vi "Autoshift.vi"() -> ()   [LabVIEW 2017]
uses:
  <vilib>/Rock Robotics/WPI/Solenoid/WPI_SolenoidDevRef.ctl
  <vilib>/Rock Robotics/WPI/Solenoid/WPI_SolenoidChannel.ctl
  <vilib>/Rock Robotics/WPI/Solenoid/WPI_SolenoidValue.ctl
  <vilib>/Rock Robotics/WPI/ThirdParty/Sensors/navX/_TypeDefs/FRIC_navX_DeviceNumbersTypeDef.ctl
  <vilib>/Rock Robotics/WPI/Utilities/WPI_GetSetVariantRefNum.vi
  <vilib>/Rock Robotics/WPI/ThirdParty/Phoenix-LabVIEW/Motor Controller/Get/CTRE_Phoenix_MotorController_GetSelectedSensorData.vi
panel:
  in  "refnum name 3":string="My Motor RefNum"
  in  "refnum name 2":string="My Motor RefNum"
  in  "refnum name":string="My Joystick RefNum"
  in  "ShifterRef":T1={"DevStatus"={"status"=FALSE, "code"=0, "source"=""}, "Pneumatics Control Module"=0, "Forward Solenoid Channel"=enum."Invalid", "Reverse Solenoid Channel"=enum."Invalid"}
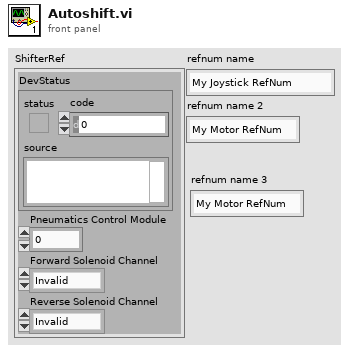
[diagram p1: front panel]
types:
  T1 = typedef "WPI_SolenoidDevRef.ctl" = cluster{"DevStatus":errorcluster, "Pneumatics Control Module":u8, "Forward Solenoid Channel":T2, "Reverse Solenoid Channel":T2}
  T2 = typedef "WPI_SolenoidChannel.ctl" = enum8{"Solenoid 0", "Solenoid 1", "Solenoid 2", "Solenoid 3", "Solenoid 4", "Solenoid 5", "Solenoid 6", "Solenoid 7", "Invalid"}
  T3 = typedef "FRIC_navX_DeviceNumbersTypeDef.ctl" = enum16{"Dev0", "Dev1", "Dev2", "Dev3"}
  T4 = typedef "WPI_SolenoidValue.ctl" = enum16{"Off", "On", "Forward", "Reverse"}
  T5 = typedef "WPI_MotorControlDeviceRef.ctl" = cluster{"DeviceStatus":errorcluster, "Type":T6, "PWM":cluster{"PWM Channel":T7, "DeadBand":T8}, "CAN":cluster{"Device Number":u8, "SetOutput VI Ref":variant, "GetOutput VI Ref":variant, "Enable VI Ref":variant, "Disable VI Ref":variant, "Data":variant}, "Invert":bool, "DIO PWM":cluster{"PWM \"Enable\" Channel":T7, "DIOChannel":T9, "PWM Rate":dbl}}
  T6 = typedef "WPI_MotorControlType.ctl" = enum16{"PWM", "CAN", "DIO PWM"}
  T7 = typedef "FPGA_DIOPWMChannel.ctl" = enum8{"PWM 0", "PWM 1", "PWM 2", "PWM 3", "PWM 4", "PWM 5", "PWM 6", "PWM 7", "PWM 8", "PWM 9", "PWM MXP 0", "PWM MXP 1", "PWM MXP 2", "PWM MXP 3", "PWM MXP 4", "PWM MXP 5", "PWM MXP 6", "PWM MXP 7", "PWM MXP 8", "PWM MXP 9", "Invalid"}
  T8 = typedef "WPI_PWMDeadband.ctl" = cluster{"Name":string, "maxPositivePwm":i32, "minPositivePwm":i32, "centerPwm":i32, "maxNegativePwm":i32, "minNegativePwm":i32, "angularRange":u16}
  T9 = typedef "FPGA_DIOChannel.ctl" = enum8{"DIO 0", "DIO 1", "DIO 2", "DIO 3", "DIO 4", "DIO 5", "DIO 6", "DIO 7", "DIO 8", "DIO 9", "DIO MXP 0", "DIO MXP 1", "DIO MXP 2", "DIO MXP 3", "DIO MXP 4", "DIO MXP 5", "DIO MXP 6", "DIO MXP 7", "DIO MXP 8", "DIO MXP 9", "DIO MXP 10", "DIO MXP 11", "DIO MXP 12", "DIO MXP 13", "DIO MXP 14", "DIO MXP 15", "SPI Port CS1", "SPI Port CS2", "SPI Port CS3", "SPI Port MISO", "SPI Port MOSI", "Invalid"}
  T10 = typedef "WPI_JoystickDevRef.ctl" = cluster{"Device":T11}
  T11 = typedef "WPI_JoystickDeviceEnum.ctl" = enum16{"USB 0", "USB 1", "USB 2", "USB 3", "USB 4", "USB 5"}
  T12 = cluster{"LinearAcceleration X":dbl, "LinearAcceleration Y":dbl, "LinearAcceleration Z":dbl}
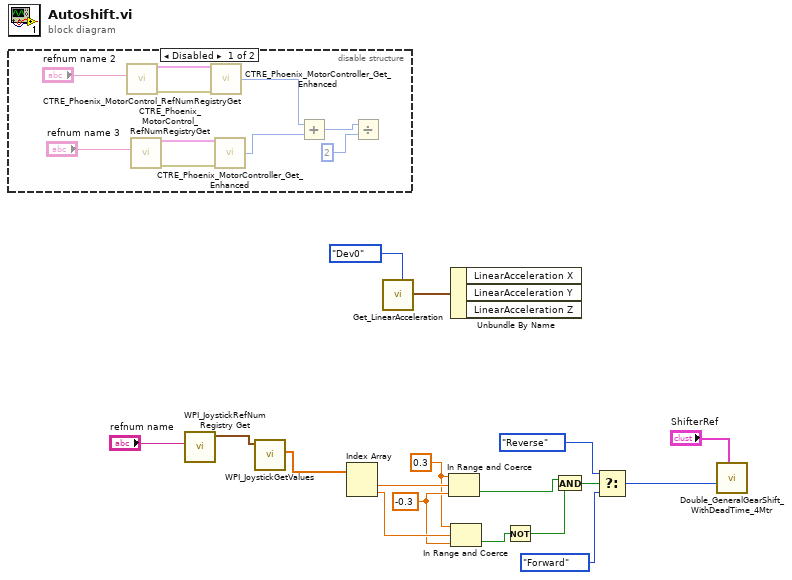
[diagram p0: block diagram]
diagram:
  w11 = -0.3 ("lower limit")
  w10 = 0.3 ("upper limit")
  n1 = disable-structure shown="Disabled" {
    frame Disabled {
      n2 = call <vilib>:"CTRE_Phoenix_MotorControl_RefNumRegistryGet.vi"("refnum name"="refnum name 2") -> ("error out"=w26:errorcluster, "PhoenixMotorControlDevRef"=w27:T5)  [unwired: 9 in]
      n3 = call <vilib>:"CTRE_Phoenix_MotorControl_RefNumRegistryGet.vi"("refnum name"="refnum name 3") -> ("error out"=w23:errorcluster, "PhoenixMotorControlDevRef"=w22:T5)  [unwired: 9 in]
      n4 = call-poly <vilib>:"CTRE_Phoenix_MotorController_Get_Enhanced.vi"("PhoenixMotorControlDevRef"=w27, "error in"=w26) -> ("Velocity (Raw Sensor Units per 100 ms)"=w21:i32)  [unwired: 10 in, 3 out]
      n5 = call-poly <vilib>:"CTRE_Phoenix_MotorController_Get_Enhanced.vi"("PhoenixMotorControlDevRef"=w22, "error in"=w23) -> ("Velocity (Raw Sensor Units per 100 ms)"=w20:i32)  [unwired: 10 in, 3 out]
      n6 = Add(x=w21, y=w20) -> (x+y=w19:i32)
      n7 = Divide(x=w19, y=2) -> ()  [unwired: 1 out]
    }
    frame Enabled {
    }
  }
  n8 = call <vilib>:"WPI_JoystickRefNum Registry Get.vi"("refnum name"="refnum name") -> ("JoystickDevRef"=w16:T10)  [unwired: 9 in, 1 out]
  n9 = call <vilib>:"WPI_JoystickGetValues.vi"("JoystickDevRef"=w16) -> ("Axes"=w14:dbl[])  [unwired: 6 in, 4 out]
  n10 = Index Array(array=w14) -> (element #1=w13:dbl, element #2=w12:dbl)  [unwired: 2 in]
  n11 = call <vilib>:"Get_LinearAcceleration.vi"("Device Number"=FRIC_navX_DeviceNumbersTypeDef."Dev0") -> ("Linear Acceleration"=w1:T12)  [unwired: 10 in]
  n12 = In Range and Coerce(upper limit=w10, x=w13, lower limit=w11) -> (In Range?=w8:bool)  [unwired: 1 out]
  n13 = Unbundle By Name(w1) -> ()  [unwired: 3 out]
  n14 = In Range and Coerce(upper limit=w10, x=w12, lower limit=w11) -> (In Range?=w9:bool)  [unwired: 1 out]
  n15 = Not(x=w9) -> (.not. x?=w7:bool)
  n16 = And(x=w8, y=w7) -> (x .and. y?=w6:bool)
  n17 = Select(t=WPI_SolenoidValue."Reverse" ("Shift Value"), s=w6, f=WPI_SolenoidValue."Forward" ("Shift Value")) -> (s? t:f=w3:T4)
  n18 = call "Double_GeneralGearShift_WithDeadTime_4Mtr.vi"("ShifterRef"="ShifterRef", "Shift Value"=w3) -> ()  [unwired: 6 in, 4 out]
